vi "read actual configuration.vi"(8 "error in":errorcluster, 11 "Scan Engine editor node in":refnum<class "Scan Engine editor node.lvclass">) -> (0 "error out":errorcluster, 2 "Scan Engine configuration out":refnum<class "Scan Engine configuration.lvclass">, 3 "Scan Engine editor node out":refnum<class "Scan Engine editor node.lvclass">)   [LabVIEW 2013, in "Scan Engine editor node.lvclass"]
uses:
  Scan Engine editor node.lvclass
  <vilib>/NI/TBM Modules/variable/module/configuration/Scan Engine configuration.lvclass
  <vilib>/NI/Tag Bus Data Framework/Configuration Editor/Classes/Module editor node/Read Module Configuration.vi
  <vilib>/NI/Tag Bus Data Framework/Configuration Editor/Classes/Module editor node/Write Module Configuration.vi
  <vilib>/NI/Tag Bus Module Framework/module configuration/TBM module configuration.lvclass
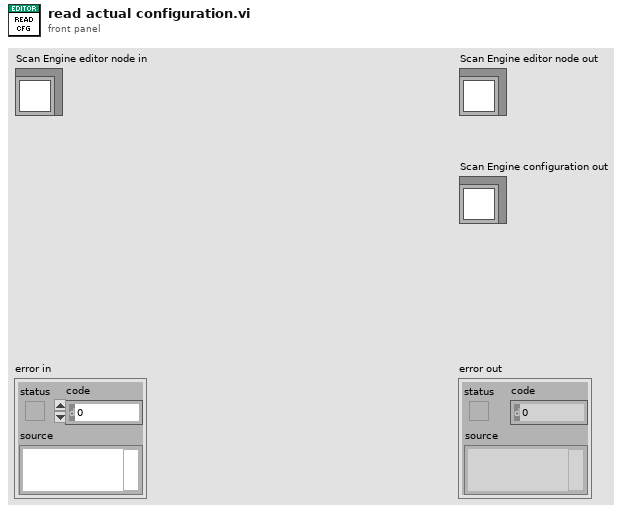
[diagram p1: front panel]
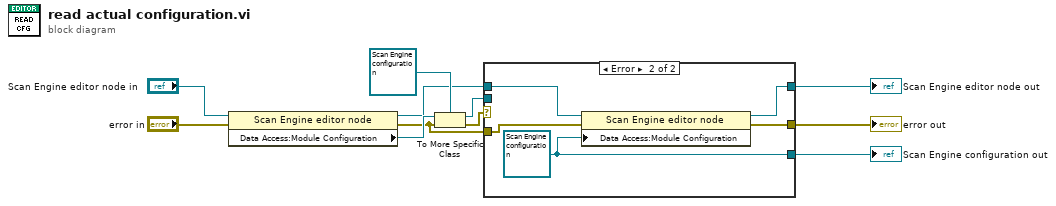
[diagram p0: block diagram]
diagram:
  n1 = property class="Scan Engine editor node"(reference="Scan Engine editor node in", error in="error in") -> (reference out=w2:refnum<class "Scan Engine editor node.lvclass">, error out=w1:errorcluster, "Data Access:Module Configuration"=w6:refnum<class "TBM module configuration.lvclass">)
  n2 = To More Specific Class(target class=refnum<class "Scan Engine configuration.lvclass"> refnum ("tag bus configurable plugin module configuration"), reference=w6, error in=w1) -> (specific class reference=w3:refnum<class "Scan Engine configuration.lvclass">, error out=w4:errorcluster)
  n3 = case shown="Error" w4 {
    selector: w4 -> [w13 _]
    tunnel: [w14 w15] -> w9
    tunnel: w3 -> [w14 _]
    tunnel: [w13 w17] -> w7
    tunnel: [w12 w16] -> w10
    tunnel: w2 -> [w12 w19]
    tunnel: w1 -> [_ w18]
    frame No Error {
    }
    frame Error {
      w15 = refnum<class "Scan Engine configuration.lvclass"> refnum ("tag bus configurable plugin module configuration")
      n4 = property class="Scan Engine editor node"(reference=w19, error in=w18, "Data Access:Module Configuration"=w15) -> (reference out=w16:refnum<class "Scan Engine editor node.lvclass">, error out=w17:errorcluster)
    }
  }
  "error out" <- w7
  "Scan Engine editor node out" <- w10
  "Scan Engine configuration out" <- w9
